vi "asynch_background_timing_pb.vi"(1 "PB Ch for Zeeman Coil Current":i32=19, 2 "Exposure Mode":u16(ring)=1 items=["Asynch shutter", "Double shot", "Video mode", "Auto exposure"], 3 "PulseBlaster Array of Arrays In":T1(array[cluster])=[{"Data Field"=0, "Delay"=0.005, "OP code"=8, "Output Bits"=[FALSE, TRUE, FALSE, FALSE, FALSE, TRUE, FALSE, FALSE, FALSE, FALSE, FALSE, FALSE, FALSE, FALSE, FALSE, FALSE, FALSE, FALSE, FALSE, FALSE, FALSE, FALSE, FALSE, FALSE], "String"="cool mot coils"}, {"Data Field"=300, "Delay"=0.000999, "OP code"=2, "Output Bits"=[FALSE, TRUE, FALSE, FALSE, FALSE, TRUE, FALSE, FALSE, FALSE, FALSE, FALSE, FALSE, FALSE, FALSE, FALSE, FALSE, FALSE, FALSE, FALSE, FALSE, FALSE, FALSE, FALSE, FALSE], "String"="mot load loop"}, {"Data Field"=1, "Delay"=1e-06, "OP code"=3, "Output Bits"=[FALSE, TRUE, FALSE, FALSE, FALSE, TRUE, FALSE, FALSE, FALSE, FALSE, FALSE, FALSE, FALSE, FALSE, FALSE, FALSE, FALSE, FALSE, FALSE, FALSE, FALSE, FALSE, FALSE, FALSE, FALSE], "String"=""}, {"Data Field"=0, "Delay"=0.001, "OP code"=0, "Output Bits"=[FALSE, TRUE, FALSE, FALSE, FALSE, TRUE, TRUE, FALSE, FALSE, FALSE, FALSE, FALSE, FALSE, FALSE, FALSE, FALSE, FALSE, FALSE, FALSE, FALSE, FALSE, FALSE, FALSE, FALSE], "String"=""}, {"Data Field"=2, "Delay"=0.000999, "OP code"=2, "Output Bits"=[FALSE, TRUE, FALSE, FALSE, FALSE, TRUE, TRUE, FALSE, FALSE, FALSE, FALSE, FALSE, FALSE, FALSE, FALSE, FALSE, FALSE, FALSE, FALSE, FALSE, FALSE, FALSE, FALSE, FALSE], "String"="mot decay loop"}, {"Data Field"=4, "Delay"=1e-06, "OP code"=3, "Output Bits"=[FALSE, TRUE, FALSE, FALSE, FALSE, TRUE, TRUE, FALSE, FALSE, FALSE, FALSE, FALSE, FALSE, FALSE, FALSE, FALSE, FALSE, FALSE, FALSE, FALSE, FALSE, FALSE, FALSE, FALSE], "String"=""}, {"Data Field"=0, "Delay"=0.04, "OP code"=0, "Output Bits"=[FALSE, TRUE, FALSE, FALSE, FALSE, TRUE, TRUE, FALSE, FALSE, FALSE, FALSE, FALSE, FALSE, FALSE, FALSE, FALSE, FALSE, FALSE, FALSE, FALSE, FALSE, FALSE, FALSE, FALSE], "String"=""}, {"Data Field"=0, "Delay"=0.00865, "OP code"=0, "Output Bits"=[FALSE, TRUE, FALSE, FALSE, FALSE, FALSE, TRUE, FALSE, FALSE, FALSE, FALSE, FALSE, FALSE, FALSE, FALSE, FALSE, FALSE, FALSE, FALSE, FALSE, FALSE, FALSE, FALSE, FALSE], "String"=""}, {"Data Field"=0, "Delay"=0.004, "OP code"=0, "Output Bits"=[FALSE, TRUE, FALSE, FALSE, FALSE, FALSE, TRUE, FALSE, FALSE, FALSE, FALSE, FALSE, FALSE, FALSE, FALSE, FALSE, FALSE, FALSE, FALSE, FALSE, FALSE, FALSE, FALSE, FALSE], "String"=""}, {"Data Field"=0, "Delay"=0.0045, "OP code"=0, "Output Bits"=[FALSE, TRUE, FALSE, FALSE, FALSE, FALSE, TRUE, FALSE, FALSE, FALSE, FALSE, FALSE, FALSE, FALSE, FALSE, FALSE, FALSE, FALSE, FALSE, FALSE, FALSE, FALSE, FALSE, FALSE], "String"="Blue MOT Cooling Time"}, {"Data Field"=0, "Delay"=5e-05, "OP code"=0, "Output Bits"=[FALSE, TRUE, FALSE, FALSE, FALSE, FALSE, TRUE, FALSE, FALSE, FALSE, FALSE, FALSE, FALSE, FALSE, FALSE, FALSE, FALSE, FALSE, FALSE, FALSE, FALSE, FALSE, FALSE, FALSE], "String"="Red MOT Cooling Time =="}, {"Data Field"=0, "Delay"=0.01, "OP code"=0, "Output Bits"=[FALSE, TRUE, FALSE, FALSE, FALSE, FALSE, TRUE, FALSE, FALSE, FALSE, FALSE, FALSE, FALSE, FALSE, FALSE, FALSE, FALSE, FALSE, FALSE, FALSE, FALSE, FALSE, FALSE, FALSE], "String"="PAS Beam with RED MOT            DELAY TIME BEFORE INTERAC"}, {"Data Field"=0, "Delay"=0.005, "OP code"=0, "Output Bits"=[FALSE, TRUE, FALSE, FALSE, TRUE, FALSE, TRUE, FALSE, FALSE, FALSE, FALSE, FALSE, FALSE, FALSE, FALSE, FALSE, FALSE, FALSE, FALSE, FALSE, FALSE, FALSE, FALSE, FALSE], "String"="image 12 delay (150n=90ndelay) INTERAC TIME"}, {"Data Field"=0, "Delay"=5e-05, "OP code"=0, "Output Bits"=[FALSE, TRUE, FALSE, FALSE, TRUE, FALSE, TRUE, FALSE, FALSE, FALSE, FALSE, FALSE, FALSE, FALSE, FALSE, FALSE, FALSE, FALSE, FALSE, FALSE, FALSE, FALSE, FALSE, FALSE], "String"="image beam on"}, {"Data Field"=0, "Delay"=0.0002, "OP code"=0, "Output Bits"=[FALSE, TRUE, FALSE, FALSE, FALSE, FALSE, TRUE, FALSE, FALSE, FALSE, FALSE, FALSE, FALSE, FALSE, FALSE, FALSE, FALSE, FALSE, FALSE, FALSE, FALSE, FALSE, FALSE, FALSE], "String"="camera minimum exposure time"}, {"Data Field"=0, "Delay"=0.07, "OP code"=0, "Output Bits"=[FALSE, TRUE, FALSE, FALSE, FALSE, FALSE, TRUE, FALSE, FALSE, FALSE, FALSE, FALSE, FALSE, FALSE, FALSE, FALSE, FALSE, FALSE, FALSE, FALSE, FALSE, FALSE, FALSE, FALSE], "String"="PixelFly Readout 1"}, {"Data Field"=0, "Delay"=0.005, "OP code"=0, "Output Bits"=[FALSE, TRUE, FALSE, FALSE, TRUE, FALSE, TRUE, FALSE, FALSE, FALSE, FALSE, FALSE, FALSE, FALSE, FALSE, FALSE, FALSE, FALSE, FALSE, FALSE, FALSE, FALSE, FALSE, FALSE], "String"="shutter opening time"}, {"Data Field"=0, "Delay"=0.0002, "OP code"=0, "Output Bits"=[FALSE, TRUE, FALSE, FALSE, FALSE, FALSE, TRUE, FALSE, FALSE, FALSE, FALSE, FALSE, FALSE, FALSE, FALSE, FALSE, FALSE, FALSE, FALSE, FALSE, FALSE, FALSE, FALSE, FALSE], "String"="Pixelfly exposure 2"}, {"Data Field"=0, "Delay"=0.07, "OP code"=0, "Output Bits"=[FALSE, TRUE, FALSE, FALSE, FALSE, FALSE, TRUE, FALSE, FALSE, FALSE, FALSE, FALSE, FALSE, FALSE, FALSE, FALSE, FALSE, FALSE, FALSE, FALSE, FALSE, FALSE, FALSE, FALSE], "String"="PixelFly readout 2"}, {"Data Field"=0, "Delay"=0.001, "OP code"=6, "Output Bits"=[FALSE, TRUE, FALSE, FALSE, FALSE, FALSE, TRUE, FALSE, FALSE, FALSE, FALSE, FALSE, FALSE, FALSE, FALSE, FALSE, FALSE, FALSE, FALSE, FALSE, FALSE, FALSE, FALSE, FALSE], "String"=""}] {"OP code" items=["Continue", "Stop", "Loop", "End Loop", "Jump", "Return", "Go To", "Long Delay", "Wait"]; "Delay" format="%.3p"}) -> (0 "PB Array of Arrays Out":T1(array[cluster]) {"OP code" items=["Continue", "Stop", "Loop", "End Loop", "Jump", "Return", "Go To", "Long Delay", "Wait"]; "Delay" format="%.2p"})   [LabVIEW 2013]
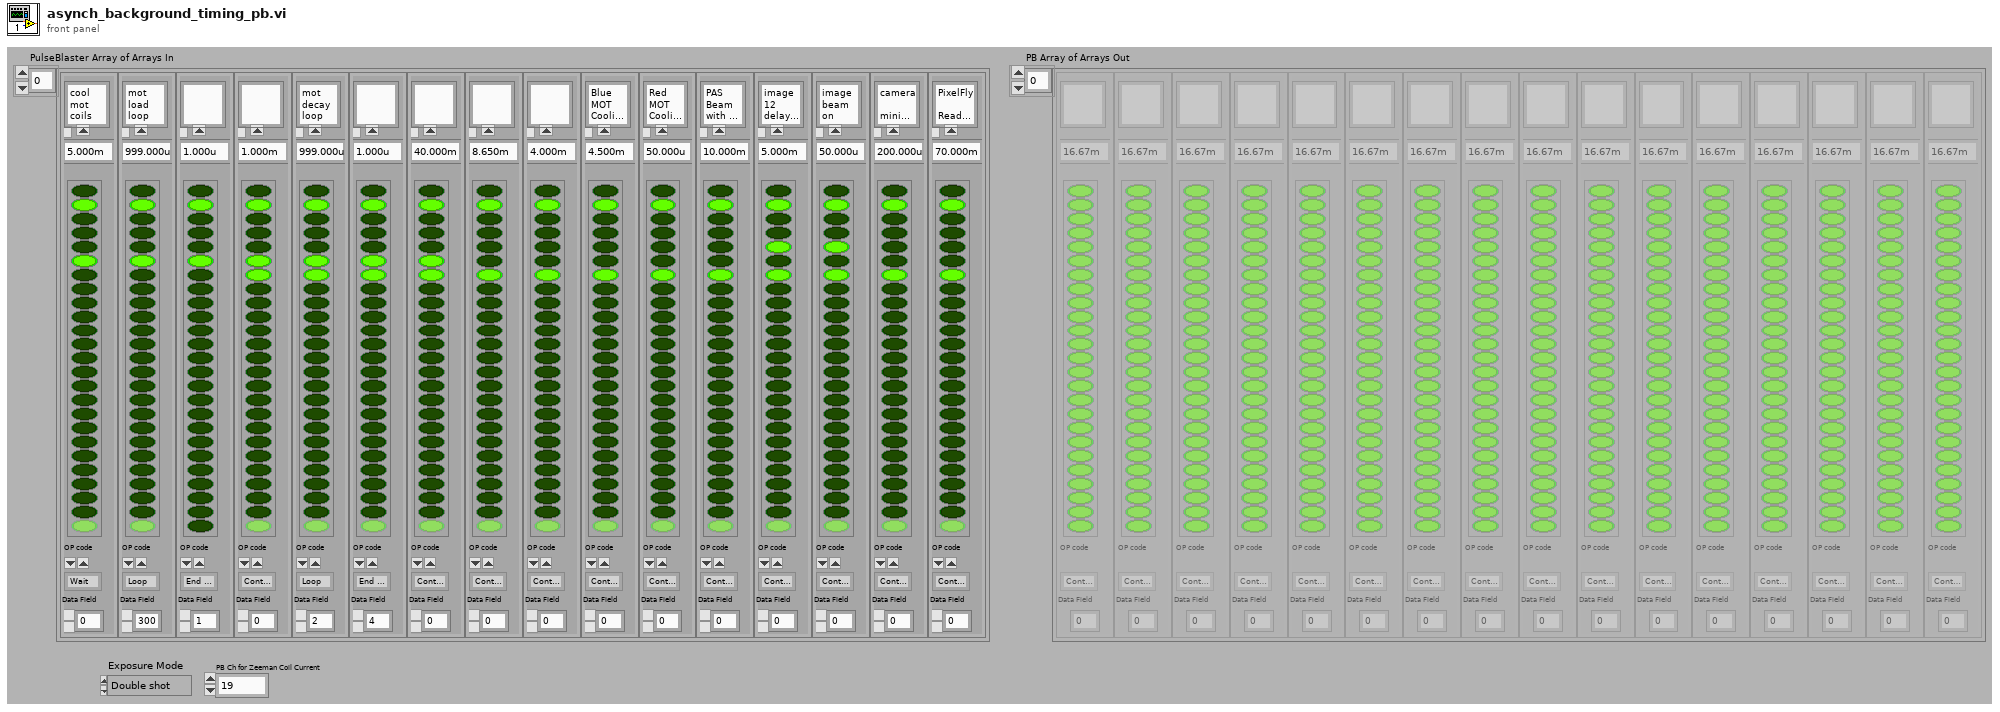
[diagram p1: front panel]
types:
  T1 = cluster{"Data Field":u32, "Delay":dbl, "OP code":u8, "Output Bits":bool[], "String":string}[]
  T2 = cluster{"Data Field":u32, "Delay":dbl, "OP code":u8, "Output Bits":bool[], "String":string}
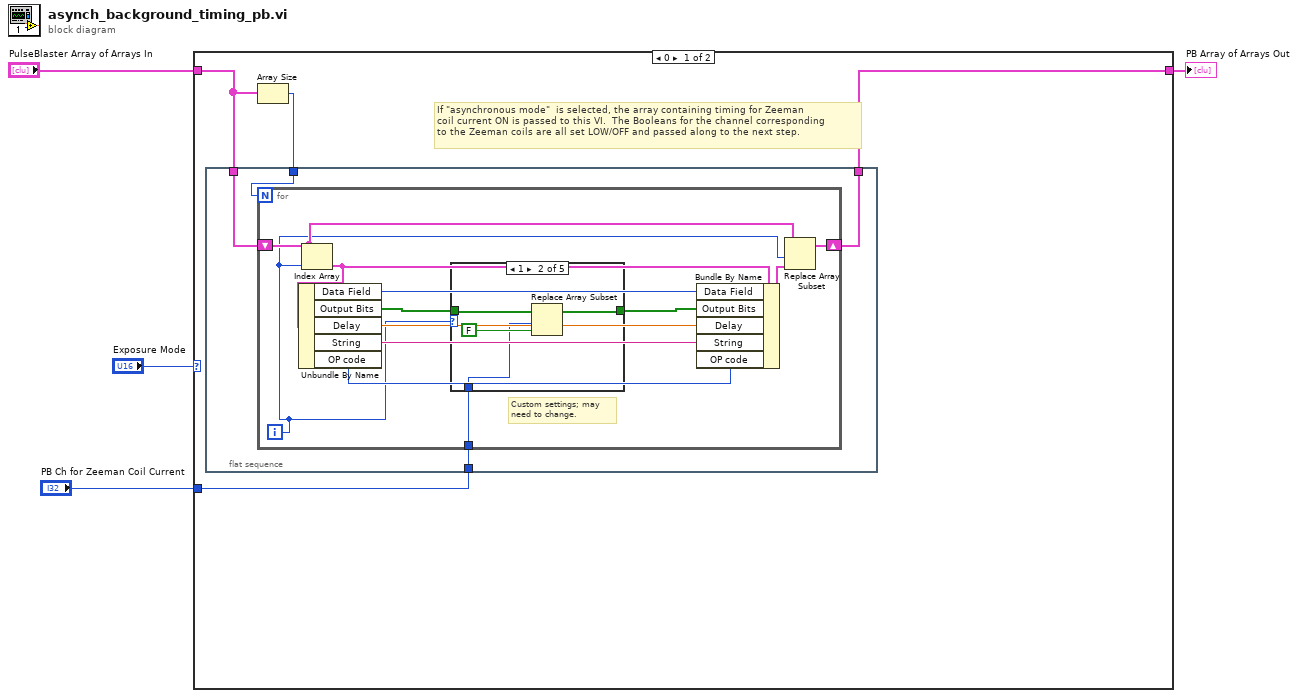
[diagram p0: block diagram]
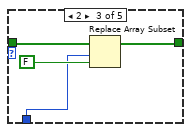
[diagram p3: hidden frame]
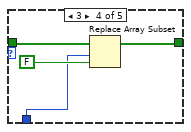
[diagram p4: hidden frame]
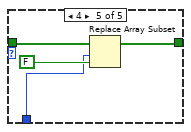
[diagram p5: hidden frame]
diagram:
  n1 = case shown="0" "Exposure Mode" {
    tunnel: "PulseBlaster Array of Arrays In" -> [w6 w42]
    tunnel: [w8 w42] -> w3
    tunnel: "PB Ch for Zeeman Coil Current" -> [w7 _]
    frame 0 {
      # "If \"asynchronous mode\"  is selected, the array containing timing for Zeeman\ncoil current ON is passed to this VI.  The Booleans for the channel corresponding\nto the Zeeman coils are all set LOW/OFF and passed along to the next step."
      n2 = flat-sequence {
        tunnel: [w12] -> w8
        tunnel: w7 -> [w11]
        tunnel: w6 -> [w10]
        tunnel: w5 -> [w9]
        frame #0 {
          n3 = for {
            N: w9 -> [_]
            shift-right: [w17] -> w12
            shift-left: w10 -> [w19]
            tunnel: w11 -> [w15]
            i -> [w13]
            # "Custom settings; may\nneed to change."
            n4 = Index Array(array=w19, index=w13) -> (element=w20:T2)
            n5 = Unbundle By Name(w20) -> ("Data Field"=w21:u32, "Output Bits"=w16:bool[], "Delay"=w18:dbl, "String"=w24:string, "OP code"=w23:u8)
            n6 = case shown="1" w13 {
              tunnel: w16 -> [w25 w29 w33 w37 w41]
              tunnel: [w25 w28 w32 w36 w40] -> w14
              tunnel: w15 -> [_ w26 w30 w34 w38]
              frame 0, Default {
                # "If for some reason stuff\ndoes not work, just pass\nalong what's already\nthere."
              }
              frame 1 {
                n7 = Replace Array Subset(array=w29, new element=FALSE ("new element/subarray"), index=w26) -> (w28:bool[])
              }
              frame 2 {
                n8 = Replace Array Subset(array=w33, new element=FALSE ("new element/subarray"), index=w30) -> (w32:bool[])
              }
              frame 3 {
                n9 = Replace Array Subset(array=w37, new element=FALSE ("new element/subarray"), index=w34) -> (w36:bool[])
              }
              frame 4 {
                n10 = Replace Array Subset(array=w41, new element=FALSE ("new element/subarray"), index=w38) -> (w40:bool[])
              }
            }
            n11 = Bundle By Name(cluster=w20, "Data Field"=w21, "Output Bits"=w14, "Delay"=w18, "String"=w24, "OP code"=w23) -> (w22:T2)
            n12 = Replace Array Subset(array=w19, new element=w22, index=w13) -> (w17:T1)
          }
        }
      }
      n13 = Array Size(array=w6) -> (size(s)=w5:i32)
    }
    frame 1, Default {
      # "Default is having Zeeman coil current ON.  The timing on the front panel\nof the PB stays just as it is programmed."
    }
  }
  "PB Array of Arrays Out" <- w3
